vi "Set Operation.vi"(8 "error in (no error)":errorcluster, 9 "Data":variant, 10 "Operation Target":u32, 11 "FPGA Reference in":refnum<class "FPGA Reference.lvclass">) -> (0 "error out":errorcluster, 3 "FPGA Reference out":refnum<class "FPGA Reference.lvclass">)   [LabVIEW 2019, in "FPGA Reference.lvclass"]
uses:
  FPGA Reference.lvclass
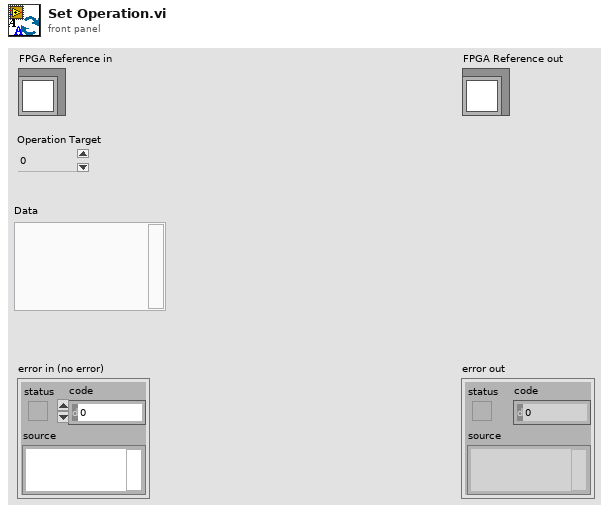
[diagram p1: front panel]
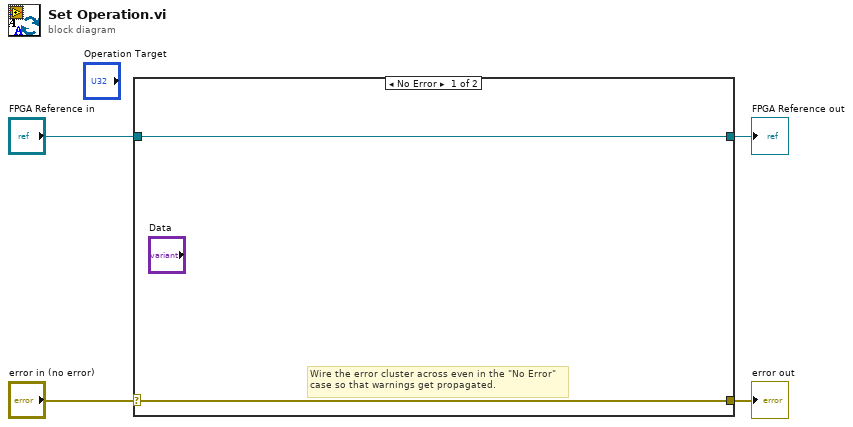
[diagram p0: block diagram]
diagram:
  n1 = case shown="No Error" "error in (no error)" {
    selector: "error in (no error)" -> [w5 w8]
    tunnel: [w5 w8] -> w3
    tunnel: [w6 w7] -> w1
    tunnel: "FPGA Reference in" -> [w6 w7]
    frame No Error {
      # "Wire the error cluster across even in the \"No Error\"\ncase so that warnings get propagated."
    }
    frame Error {
    }
  }
  "error out" <- w3
  "FPGA Reference out" <- w1
